vi "Get Board Size.vi"() -> (3 "Board Size":cluster{"Width":u32, "Height":u32})   [LabVIEW 2019]
doc: "Returns the size of the board for the Battleships game."
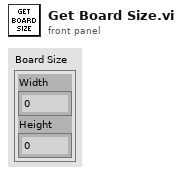
[diagram p1: front panel]
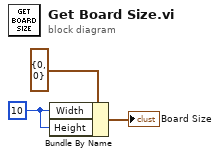
[diagram p0: block diagram]
diagram:
  w1 = u32 10
  n1 = Bundle By Name(cluster=cluster{"Width":u32, "Height":u32} {"Width"=0, "Height"=0} ("Board Size"), "Width"=w1, "Height"=w1) -> (→"Board Size":cluster{"Width":u32, "Height":u32})
